vi "UE9 PWM, FirmCounter, and Counter Example.vi"(8 "error in":errorcluster, 9 "PWM Duty Cycle [%]":dbl=50.0 format="%.1f", 10 "PWM Frequency [Hz]":dbl=1000.0 format="%.1f") -> (0 "error out":errorcluster, 2 "Actual Frequency":dbl format="%.1f")   [LabVIEW 2021]
panel:
  in  "Case Constant\n(See Context Help)":bool=TRUE
  out "Counter0":u32
  out "Timer Value Reads":u32[](array[numeric])
  in  "FirstFound":bool=TRUE
  in  "Address":string="1"
  in  "ConnectionType":u16(ring) items=["LJ_ctUSB", "LJ_ctETHERNET"]
  out "PWM Timer Value":u16
  in  "milliseconds to count":u32=1000
  in  "# of firm counters to enable":u32=2
  out "TimerClockDivisor":u8
  out "TimerClockBase":string
  out "Error Message":string
  # "Demonstrates 1 channel of 8-bit PWM output, 1-5 firmware counters, and 1 hardware counter.  Short FIO0 (PWM output)\nto FIO1-FIO5 (firmcounters) and next available FIO (hardware counter).  Enables PWM, then counts for the specified amount\nof time, then reads the counts, then disables PWM.\nAssumes Control power level is at the default level of \"High\" (Control firmware 1.08 or higher).\nTimer clock, and timer clock divisor, are chosen to get as close as possible to the desired PWM frequency.\nFor 660<=f<=187500, system clock is used for timer clock.\nFor f<660, fixed 750kHz timer clock is used for timer clock."
  # "PWM reads 0"
  # "187500 Hz max, 11.4 Hz min"
  # "First firm counter"
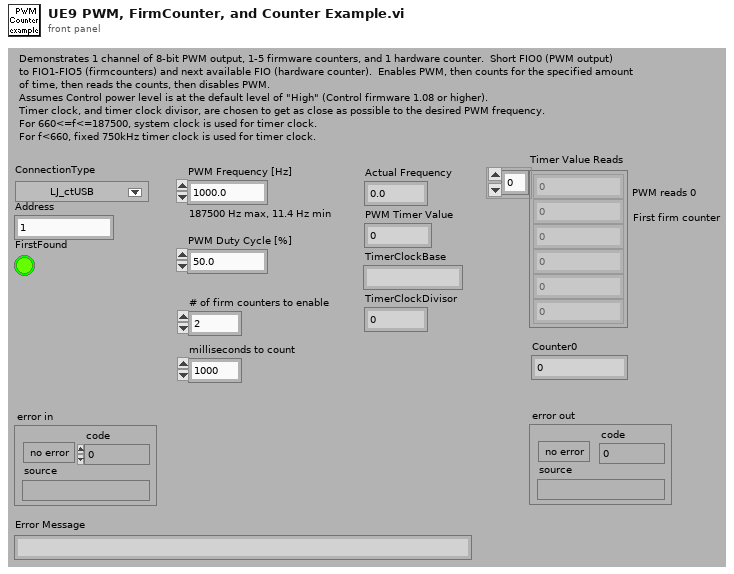
[diagram p1: front panel]
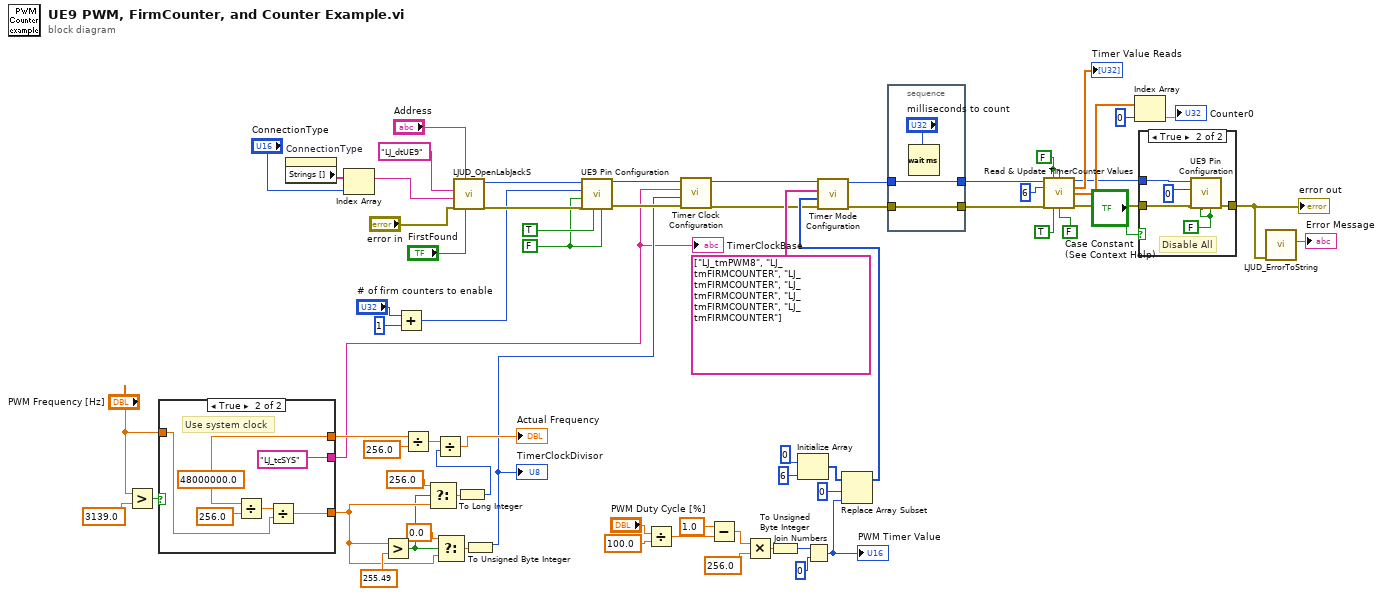
[diagram p0: block diagram]
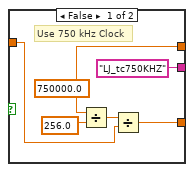
[diagram p3: hidden frame]
diagram:
  w11 = FALSE ("Enable Counter0")
  w43 = FALSE ("Reset Counter0")
  n1 = Greater?(x="PWM Frequency [Hz]", y=3139.0) -> (0:w49:bool)
  n2 = case shown="True" w49 {
    tunnel: "PWM Frequency [Hz]" -> [w72 w78]
    tunnel: [w71 w77] -> w24
    tunnel: [w70 w76] -> w61
    tunnel: ["LJ_tc750KHZ" "LJ_tcSYS"] -> w3
    frame False {
      w70 = 750000.0 ("x")
      # "Use 750 kHz Clock"
      n3 = Divide(x=w70, y=256.0) -> (x/y=w74:dbl)
      n4 = Divide(x=w74, y=w72) -> (x/y=w71:dbl)
    }
    frame True {
      w76 = 48000000.0 ("x")
      # "Use system clock"
      n5 = Divide(x=w76, y=256.0) -> (x/y=w80:dbl)
      n6 = Divide(x=w80, y=w78) -> (x/y=w77:dbl)
    }
  }
  "TimerClockBase" <- w3
  n7 = property on="ConnectionType" class="Ring (strict)"() -> ("Strings []"=w20:string[])  [unwired: 2 in, 2 out]
  n8 = Index Array(array=w20, index="ConnectionType") -> (element=w18:string)
  n9 = Greater?(x=w24, y=255.49) -> (0:w23:bool)
  n10 = Add(x="# of firm counters to enable", y=u32 1) -> (x+y=w10:u32)
  n11 = Divide(x=w61, y=256.0) -> (x/y=w63:dbl)
  n12 = Select(t=256.0, s=w23, f=w24) -> (s? t:f=w26:dbl)
  n13 = Select(t=0.0, s=w23, f=w24) -> (s? t:f=w64:dbl)
  n14 = call "LJUD_OpenLabJackS.vi"("FirstFound"="FirstFound", "Address"="Address", "error in"="error in", "ConnectionType"=w18, "DeviceType"="LJ_dtUE9") -> ("error out"=w15:errorcluster, "Handle"=w16:i32)  [unwired: 4 in, 1 out]
  n15 = To Long Integer(number=w26) -> (32bit integer=w22:i32)
  n16 = Divide(x=w63, y=w22) -> (x/y=→"Actual Frequency":dbl)
  n17 = To Unsigned Byte Integer(number=w64) -> (unsigned 8bit integer=w4:u8)
  "TimerClockDivisor" <- w4
  n18 = call "UE9 Pin Configuration.vi"("Enable Counter1"=w11, "Enable Counter0"=TRUE, "error in"=w15, "Enable DACs"=w11, "Number of Timers Enabled"=w10, "Handle In"=w16) -> ("error out"=w7:errorcluster, "Handle Out"=w6:i32)  [unwired: 4 in]
  n19 = Divide(x="PWM Duty Cycle [%]", y=100.0) -> (x/y=w56:dbl)
  n20 = call "Timer Clock Configuration.vi"("error in"=w7, "Timer Clock Divisor"=w4, "Timer Clock Base"=w3, "Handle In"=w6) -> ("error out"=w8:errorcluster, "Handle Out"=w5:i32)  [unwired: 6 in]
  n21 = Subtract(x=1.0, y=w56) -> (x-y=w54:dbl)
  n22 = Multiply(x=w54, y=256.0) -> (x*y=w51:dbl)
  n23 = To Unsigned Byte Integer(number=w51) -> (unsigned 8bit integer=w53:u8)
  n24 = Initialize Array(u16 0 ("PWM Timer Value"), 6 ("Dimension Size")) -> (w31:u16[])
  n25 = Join Numbers(hi=w53, lo=u8 0) -> ((hi.lo)=w30:u16)
  "PWM Timer Value" <- w30
  n26 = Replace Array Subset(array=w31, new element=w30, index=0 ("Index")) -> (w9:u16[])
  n27 = call "Timer Mode Configuration.vi"("error in"=w8, "TimerValues"=w9, "TimerModes"=string[] ["LJ_tmPWM8", "LJ_tmFIRMCOUNTER", "LJ_tmFIRMCOUNTER", "LJ_tmFIRMCOUNTER", "LJ_tmFIRMCOUNTER", "LJ_tmFIRMCOUNTER"], "Handle In"=w5) -> ("error out"=w13:errorcluster, "Handle Out"=w14:i32)  [unwired: 6 in]
  n28 = stacked-sequence {
    tunnel: w13 -> [w83]
    tunnel: [w83] -> w27
    tunnel: w14 -> [w82]
    tunnel: [w82] -> w28
    frame #0 {
      n29 = Wait (ms)(milliseconds to wait="milliseconds to count") -> ()  [unwired: 1 out]
    }
  }
  n30 = call "Read & Update TimerCounter Values.vi"("Handle In"=w28, "Reset Counter0"=w43, "Reset Counter1"=w43, "# Timers to Read"=6, "error in"=w27, "Read Counter0"=TRUE ("Reset Counter0"), "Read Counter1"=FALSE ("Reset Counter0")) -> ("Handle Out"=w36:i32, "Timer Value Reads"=→"Timer Value Reads":dbl[], "Counter Value Reads"=w40:dbl[], "error out"=w37:errorcluster)  [unwired: 5 in]
  n31 = Index Array(array=w40, index=0 ("Index")) -> (element=→"Counter0":dbl)
  n32 = case shown="True" "Case Constant\n(See Context Help)" {
    tunnel: w37 -> [w84 w89]
    tunnel: w36 -> [_ w88]
    tunnel: [w84 w87] -> w35
    frame False {
    }
    frame True {
      w85 = FALSE ("Enable Counter0")
      # "Disable All"
      n33 = call "UE9 Pin Configuration.vi"("Enable Counter1"=w85, "Enable Counter0"=w85, "error in"=w89, "Number of Timers Enabled"=0 ("# Timers Enabled"), "Handle In"=w88) -> ("error out"=w87:errorcluster)  [unwired: 5 in, 1 out]
    }
  }
  "error out" <- w35
  n34 = call "LJUD_ErrorToString.vi"("error in"=w35) -> ("String"=→"Error Message":string)  [unwired: 10 in]
